vi "getValFromVariant_string.vi"(8 "error in (no error)":errorcluster, 10 "name":string, 11 "variant":variant) -> (0 "error out":errorcluster, 3 "value":string)   [LabVIEW 2018]
doc: "Get the value from variant (string)."
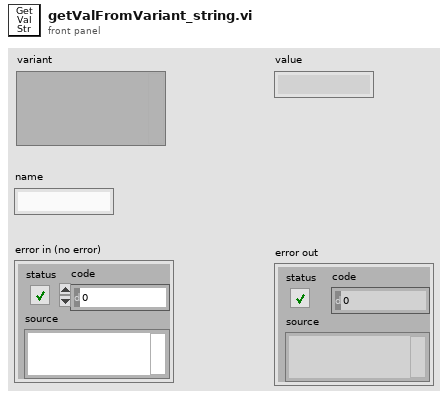
[diagram p1: front panel]
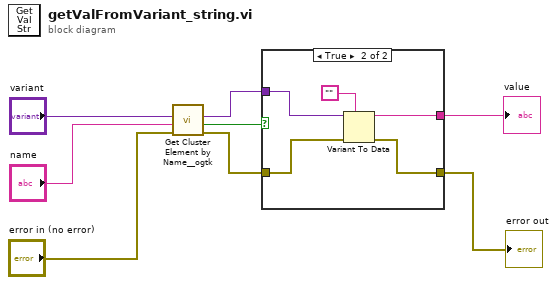
[diagram p0: block diagram]
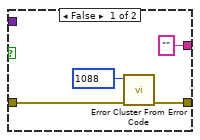
[diagram p2: hidden frame]
diagram:
  n1 = call <userlib>:"Get Cluster Element by Name__ogtk.vi"("error in (no error)"="error in (no error)", "Element Name"="name", "Cluster"="variant") -> ("error out"=w3:errorcluster, "found?"=w5:bool, "VElement"=w4:variant)  [unwired: 6 in]
  n2 = case shown="True" w5 {
    tunnel: w4 -> [_ w17]
    tunnel: w3 -> [w11 w16]
    tunnel: [w12 w15] -> w2
    tunnel: ["" w14] -> w1
    frame False {
      n3 = call <vilib>:"Error Cluster From Error Code.vi"("error in (no error)"=w11, "error code (0)"=1088) -> ("error out"=w12:errorcluster)  [unwired: 7 in]
    }
    frame True {
      n4 = Variant To Data(error in=w16, type="", Variant=w17) -> (data=w14:string, error out=w15:errorcluster)
    }
  }
  "error out" <- w2
  "value" <- w1
